vi "RSZVB Get TRM Number Of Units.vi"(8 "error in (no error)":errorcluster {"code" format="%.0x"}, 11 "VISA resource name":refnum<visa-resource-name>) -> (0 "error out":errorcluster {"code" format="%.0x"}, 2 "Number Of Units":i32, 3 "VISA resource name out":refnum<visa-resource-name>)   [LabVIEW 2011]
doc: "This VI queries the number of connected extension units R&S ZVAX-TRM. \n\nRemote-control command(s):\nSYSTem:COMMunicate:RDEVice:TEUNit:COUNt?"
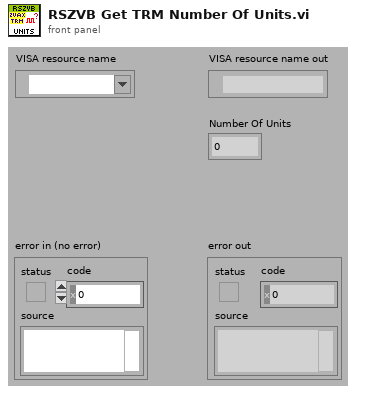
[diagram p1: front panel]
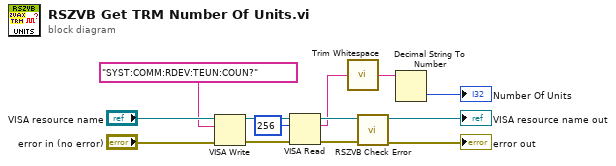
[diagram p0: block diagram]
diagram:
  n1 = VISA Write(VISA resource name="VISA resource name", write buffer="SYST:COMM:RDEV:TEUN:COUN?" ("format string"), error in (no error)="error in (no error)") -> (VISA resource name out=w13:refnum<visa-resource-name>, error out=w12:errorcluster)  [unwired: 1 out]
  n2 = VISA Read(VISA resource name=w13, byte count=u32 256, error in (no error)=w12) -> (VISA resource name out=w10:refnum<visa-resource-name>, read buffer=w9:string, error out=w11:errorcluster)  [unwired: 1 out]
  n3 = call <vilib>:"Trim Whitespace.vi"("string"=w9) -> ("trimmed string"=w1:string)  [unwired: 1 in]
  n4 = call "RSZVB Check Error.vi"("error in (no error)"=w11, "VISA session"=w10) -> ("error out"=→"error out":errorcluster, "dup VISA session"=→"VISA resource name out":refnum<visa-resource-name>)  [unwired: 8 in]
  n5 = Decimal String To Number(string=w1) -> (number=→"Number Of Units":i32)  [unwired: 2 in, 1 out]
